vi "test.vi"() -> ()   [LabVIEW 2009, in "SudukuBoard.lvclass"]
uses:
  SudukuBoard.lvclass
  SudukuState/SudukuState.lvclass
  Graph/SearchMethod.ctl
  Graph/Graph.lvclass
panel:
  out "Solution":i32[][](array[numeric])
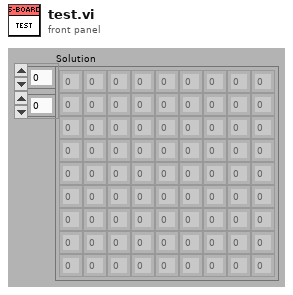
[diagram p1: front panel]
types:
  T1 = typedef "Graph.lvclass/SearchMethod.ctl" = enum16{"Breadth (First)", "Depth (First)", "Best First", "Breadth (Best)", "Depth (Best)"}
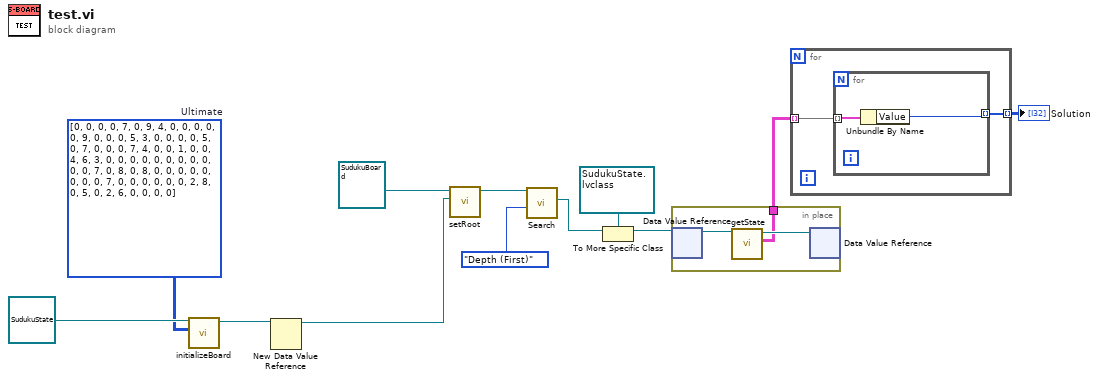
[diagram p0: block diagram]
diagram:
  w3 = i32[][] [[0, 0, 0, 0, 7, 0, 9, 4, 0], [0, 0, 0, 0, 9, 0, 0, 0, 5], [3, 0, 0, 0, 0, 5, 0, 7, 0], [0, 0, 7, 4, 0, 0, 1, 0, 0], [4, 6, 3, 0, 0, 0, 0, 0, 0], [0, 0, 0, 0, 0, 7, 0, 8, 0], [8, 0, 0, 0, 0, 0, 0, 0, 0], [7, 0, 0, 0, 0, 0, 0, 2, 8], [0, 5, 0, 2, 6, 0, 0, 0, 0]]  # Ultimate
  n1 = call "initializeBoard.vi"("Board"=w3, "SudukuState in"=refnum<class "SudukuState.lvclass"> refnum ("SudukuState.lvclass")) -> ("SudukuState out"=w2:refnum<class "SudukuState.lvclass">)  [unwired: 8 in, 1 out]
  n2 = New Data Value Reference(data value=w2) -> (data value reference=w1:refnum<data-value>)  [unwired: 1 in, 1 out]
  n3 = call "setRoot.vi"("Root"=w1, "Graph in"=refnum<class "SudukuBoard.lvclass"> refnum ("SudukuBoard.lvclass")) -> ("Graph out"=w8:refnum<class "SudukuBoard.lvclass">)  [unwired: 8 in, 1 out]
  n4 = call "Search.vi"("SearchMethod"=SearchMethod."Depth (First)", "Graph in"=w8) -> ("Node"=w11:refnum<data-value>)  [unwired: 6 in, 3 out]
  n5 = To More Specific Class(target class=refnum<data-value> refnum ("data value reference"), reference=w11) -> (specific class reference=w10:refnum<data-value>)  [unwired: 1 in, 1 out]
  n6 = in-place {
    in-place-border: [w13] -> w5
    n7 = in-place-dvr #1(w10) -> (w15:refnum<class "SudukuState.lvclass">)  [unwired: 1 out]
    n8 = call "getState.vi"("SudukuState in"=w15) -> ("State"=w13:cluster{"Value":i32, "Options":i32[]}[][], "SudukuState out"=w14:refnum<class "SudukuState.lvclass">)  [unwired: 8 in, 1 out]
    n9 = in-place-dvr #1(w14) -> ()  [unwired: 2 out]
  }
  n10 = for {
    tunnel: w5 -> [w17] mode=indexing
    tunnel: [w16] -> w4 mode=indexing
    n11 = for {
      tunnel: w17 -> [w19] mode=indexing
      tunnel: [w18] -> w16 mode=indexing
      n12 = Unbundle By Name(w19) -> ("Value"=w18:i32)
    }
  }
  "Solution" <- w4
